vi "_Advantest_Read_Value.vi"(6 "GPIB address (19)":string="2") -> (0 "error out":errorcluster, 1 "Numeric 2":i8, 2 "Numeric":dbl, 3 "Regime":string, 4 "String":string)   [LabVIEW 2013]
panel:
  in  "error in (no error)":errorcluster
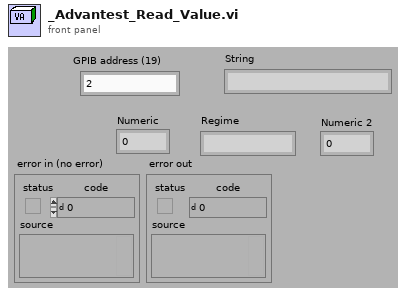
[diagram p1: front panel]
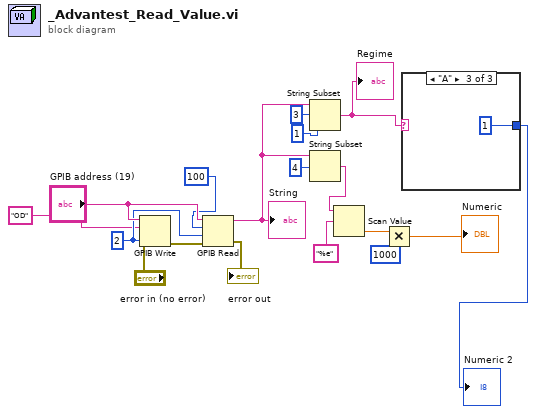
[diagram p0: block diagram]
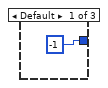
[diagram p2: hidden frame]
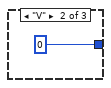
[diagram p3: hidden frame]
diagram:
  w14 = 2
  n1 = GPIB Write(0:"GPIB address (19)", 1:"OD", 2:w14, 3:"error in (no error)") -> (6:w17:errorcluster)  [unwired: 1 in, 1 out]
  n2 = GPIB Read(0:"GPIB address (19)", 1:100, 2:w14, 3:w17) -> (5:w8:string, 7:→"error out":errorcluster)  [unwired: 1 in, 1 out]
  "String" <- w8
  n3 = String Subset(string=w8, offset (0)=3, length (rest)=1) -> (substring=w2:string)
  "Regime" <- w2
  n4 = String Subset(string=w8, offset (0)=4) -> (substring=w9:string)  [unwired: 1 in]
  n5 = Scan Value(string=w9, format string="%e") -> (value=w5:dbl)  [unwired: 1 in, 1 out]
  n6 = Multiply(x=w5, y=1000) -> (x*y=→"Numeric":dbl)
  n7 = case shown="\"A\"" w2 {
    tunnel: [-1 0 1] -> w1
    frame Default {
    }
    frame "V" {
    }
    frame "A" {
    }
  }
  "Numeric 2" <- w1
